vi "9250-4.vi"() -> ()   [LabVIEW 2019]
uses:
  <vilib>/myRIO/Instrument Drivers/Onboard IO/I2C/typedefs/I2C Reference.ctl
  <vilib>/myRIO/Common/Instrument Driver Framework/Utilities/typedefs/myRIO Generic Hardware Reference.ctl
  <vilib>/myRIO/Common/Instrument Driver Framework/Utilities/typedefs/Hardware Version Enum.ctl
  <vilib>/myRIO/Common/Instrument Driver Framework/Utilities/typedefs/myRIO v1.0 Reference.ctl
  <vilib>/myRIO/Common/Instrument Driver Framework/Utilities/typedefs/Generic FPGA Reference.ctl
  <vilib>/myRIO/Common/Instrument Driver Framework/myRIO v1.0/I2C/typedefs/I2C Channels Enum.ctl
  <vilib>/myRIO/Instrument Drivers/Onboard IO/I2C/typedefs/I2C Configuration.ctl
  <vilib>/myRIO/Instrument Drivers/Onboard IO/I2C/typedefs/I2C Transfer Rate.ctl
  <vilib>/myRIO/Instrument Drivers/Onboard IO/I2C/I2C.lvlib
panel:
  out "Waveform Chart":dbl(graph)
  out "Y min value":dbl
  out "Y max value":dbl
  out "X min value":dbl
  out "X max value":dbl
  out "measure":dbl[](array[numeric])
  in  "stop":bool
  out "degree":dbl
  out "Self-test":dbl[](array[numeric])
  out "I2C Ref Out":T1={"myRIO Reference"={"myRIO Model"=enum."Unknown", "myRIO Hardware Reference"={"Generic FPGA Reference"=refnum, "Allow multiple opens"=FALSE}}, "I2C Channels Enum"=enum."Not Connected", "I2C Configuration"={"I2C Transfer Rate"=enum."Fast mode (400 kbps)"}}
  out "error out":errorcluster
  in  "Error In":errorcluster
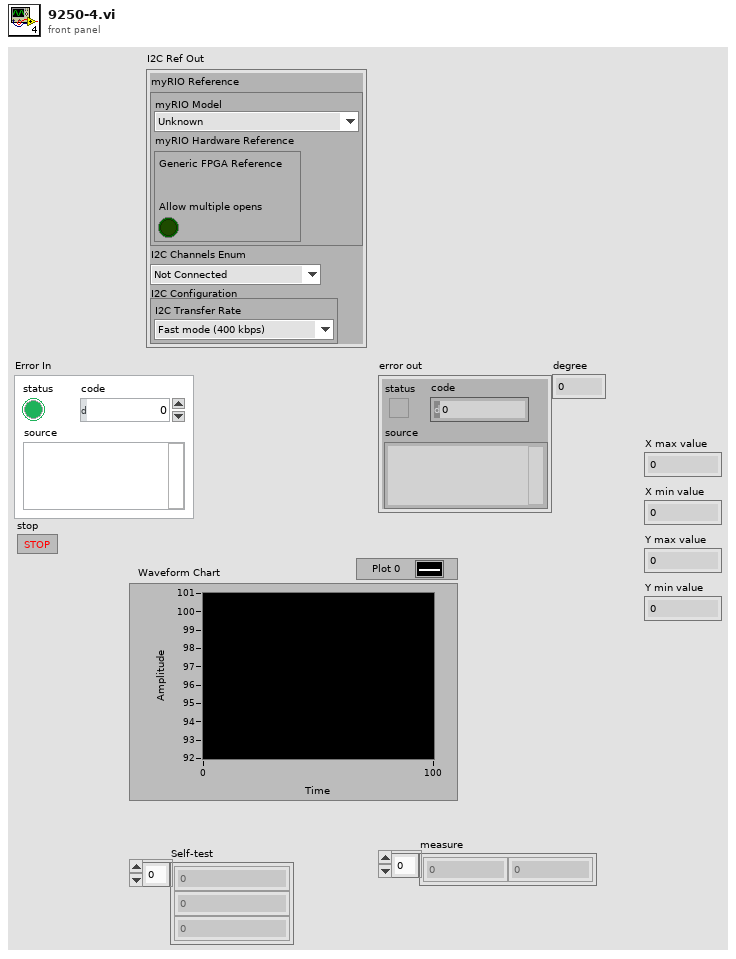
[diagram p1: front panel]
types:
  T1 = typedef "I2C.lvlib/I2C Reference.ctl" = cluster{"myRIO Reference":T2, "I2C Channels Enum":T6, "I2C Configuration":T7}
  T2 = typedef "myRIO Generic Hardware Reference.ctl" = cluster{"myRIO Model":T3, "myRIO Hardware Reference":T4}
  T3 = typedef "Hardware Version Enum.ctl" = enum16{"Unknown", "myRIO-1900", "myRIO-1950", "roboRIO", "NI ELVIS RIO CM", "ELVIS III"}
  T4 = typedef "myRIO v1.0 Reference.ctl" = cluster{"Generic FPGA Reference":T5, "Allow multiple opens":bool}
  T5 = typedef "Generic FPGA Reference.ctl" = refnum<k20>
  T6 = typedef "I2C Channels Enum.ctl" = enum16{"Not Connected", "A/I2C", "B/I2C", "I2C/I2C"}
  T7 = typedef "I2C.lvlib/I2C Configuration.ctl" = cluster{"I2C Transfer Rate":T8}
  T8 = typedef "I2C.lvlib/I2C Transfer Rate.ctl" = enum16{"Standard mode (100 kbps)", "Fast mode (400 kbps)"}
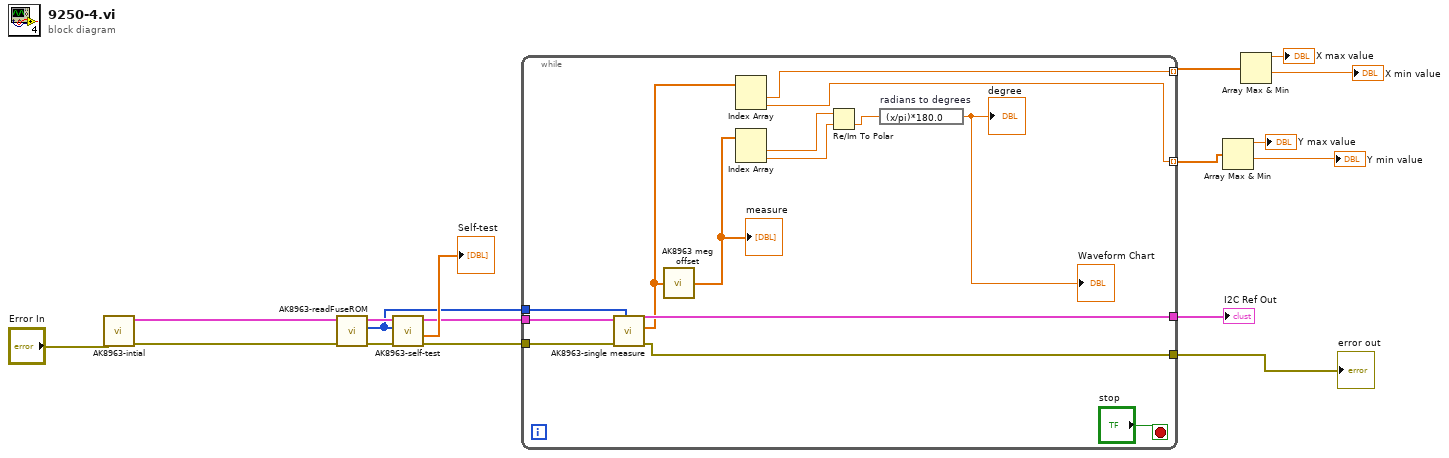
[diagram p0: block diagram]
diagram:
  n1 = call "AK8963-intial.vi"("Error In"="Error In") -> ("Error Out"=w16:errorcluster, "I2C Ref Out"=w15:T1)  [unwired: 9 in]
  n2 = call "AK8963-readFuseROM.vi"("error in (no error)"=w16, "I2C Ref In"=w15) -> ("error out"=w14:errorcluster, "ASA"=w9:u8[], "I2C Ref Out"=w13:T1)  [unwired: 7 in]
  n3 = call "AK8963-self-test.vi"("error in (no error)"=w14, "ASA"=w9, "I2C Ref In"=w13) -> ("error out"=w11:errorcluster, "Self-test"=→"Self-test":dbl[], "I2C Ref Out"=w10:T1)  [unwired: 6 in]
  n4 = while {
    tunnel: w11 -> [w31]
    tunnel: w10 -> [w30]
    tunnel: w9 -> [w29]
    tunnel: [w28] -> w8
    tunnel: [w27] -> w7
    tunnel: [w20] -> w6 mode=indexing
    tunnel: [w19] -> w1 mode=indexing
    stop <- "stop" stop-if-true
    n5 = call "AK8963-single measure.vi"("ASA"=w29, "error in (no error)"=w31, "I2C Ref In"=w30) -> ("error OUT"=w27:errorcluster, "measure"=w18:dbl[], "I2C Ref Out"=w28:T1)  [unwired: 6 in]
    n6 = call "AK8963 meg offset.vi"("measure"=w18) -> ("measure OUT"=w21:dbl[])
    "measure" <- w21
    n7 = Index Array(array=w18) -> (element #1=w20:dbl, element #2=w19:dbl)  [unwired: 2 in]
    n8 = Index Array(array=w21) -> (element #1=w24:dbl, element #2=w23:dbl)  [unwired: 2 in]
    n9 = Re/Im To Polar(2:w23, 3:w24) -> (0:w25:dbl)  [unwired: 1 out]
    n10 = expression code="(x/pi)*180.0" "radians to degrees"(w25) -> (→"degree" →"Waveform Chart":dbl)
  }
  "error out" <- w7
  "I2C Ref Out" <- w8
  n11 = Array Max & Min(array=w1) -> (max value=→"Y max value":dbl, min value=→"Y min value":dbl)  [unwired: 2 out]
  n12 = Array Max & Min(array=w6) -> (max value=→"X max value":dbl, min value=→"X min value":dbl)  [unwired: 2 out]
